vi "Manipulator Inertia Torque.vi"   [LabVIEW 2017, in "NI_Kinematics.lvlib"]
doc: "Calculates the joint torques that result from inertia given the joint accelerations you specify. Wire data to the <B>joint positions</B> input to determine the polymorphic instance to use or manually select the instance.\n\n<B>.m file:</B> itorque"
uses:
  <vilib>/robotics/Kinematics/NI_Kinematics.lvlib
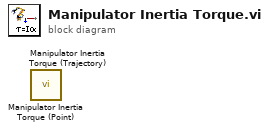
[diagram p0: block diagram]
diagram:
  n1 = call <vilib>:"Manipulator Inertia Torque (Point).vi"() -> ()  [unwired: 9 in, 3 out]
  n2 = call <vilib>:"Manipulator Inertia Torque (Trajectory).vi"() -> ()  [unwired: 9 in, 3 out]
